vi "Init.vi"(7 "Mutable (F)":bool, 8 "error in (no error)":errorcluster) -> (0 "error out":errorcluster, 3 "Config Manager out":refnum<class "Config Manager.lvclass">)   [LabVIEW 2023, in "CDM-Config.lvlib" / "Config Manager.lvclass"]
doc: "Creates a new instance of a Config ready for elements to be created in it. To load an existing config instead,initialize a Storage implementation and call its Load.vi\n\nWhen done with the Config instance, be sure to call <b>Cleanup.vi</b>"
uses:
  Config Manager.lvclass
  Ref Data.ctl
  Config Element/Config Element.lvclass
  Config Manager.lvclass/Config Manager.ctl
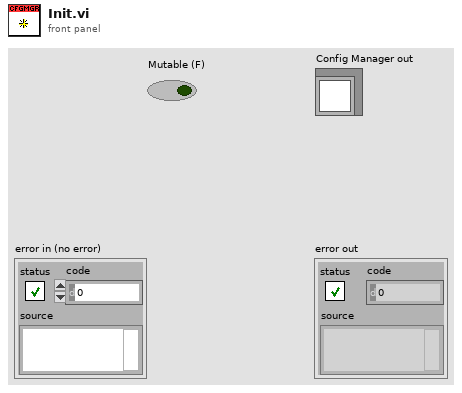
[diagram p1: front panel]
types:
  T1 = typedef "CDM-Config.lvlib/Config Manager.lvclass/Ref Data.ctl" = cluster{"Elements":refnum<class "Config Element.lvclass">[], "Hierarchy Map":map{string[], i32}, "Element Map":map{refnum<class "Config Element.lvclass">, i32}}
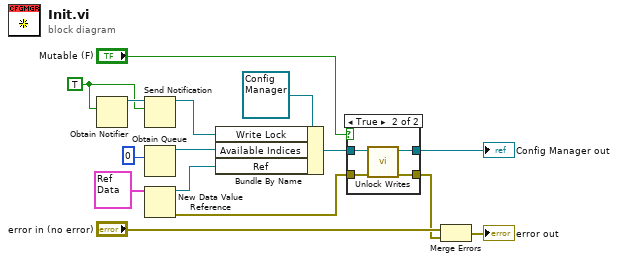
[diagram p0: block diagram]
diagram:
  w6 = TRUE
  n1 = Obtain Notifier(notification data type=w6) -> (notifier out=w7:refnum<notifier>)  [unwired: 3 in, 2 out]
  n2 = Send Notification(notification=w6, notifier=w7) -> (notifier out=w5:refnum<notifier>)  [unwired: 1 in, 1 out]
  n3 = Obtain Queue(element data type=0) -> (queue out=w8:refnum<queue>)  [unwired: 4 in, 2 out]
  n4 = New Data Value Reference(data value=T1 {"Elements"=[], "Hierarchy Map"={}, "Element Map"={}} ("Ref Data")) -> (data value reference=w13:refnum<data-value>, error out=w3:errorcluster)  [unwired: 1 in]
  n5 = Bundle By Name(cluster=refnum<class "Config Manager.lvclass"> refnum ("Config Manager in"), "Write Lock"=w5, "Available Indices"=w8, "Ref"=w13) -> (w11:refnum<class "Config Manager.lvclass">)
  n6 = case shown="True" "Mutable (F)" {
    tunnel: w11 -> [w17 w21]
    tunnel: [w17 w20] -> w4
    tunnel: w3 -> [w16 w19]
    tunnel: [w16 w18] -> w2
    frame False {
    }
    frame True {
      n7 = call "Unlock Writes.vi"("error in (no error)"=w19, "Config Manager in"=w21) -> ("error out"=w18:errorcluster, "Config Manager out"=w20:refnum<class "Config Manager.lvclass">)  [unwired: 8 in]
    }
  }
  "Config Manager out" <- w4
  n8 = Merge Errors("error in (no error)", w2) -> (→"error out":errorcluster)
